vi "Init Actor Core.vi"(8 "error in (no error)":errorcluster, 11 "App in":refnum<class "App.lvclass">) -> (0 "error out":errorcluster, 3 "App out":refnum<class "App.lvclass">)   [LabVIEW 2016, in "App.lvlib" / "App.lvclass"]
uses:
  App.lvclass
  App.lvclass/App.ctl
  Dynamic Instrument/Dynamic Instrument/Dynamic Instrument.lvclass
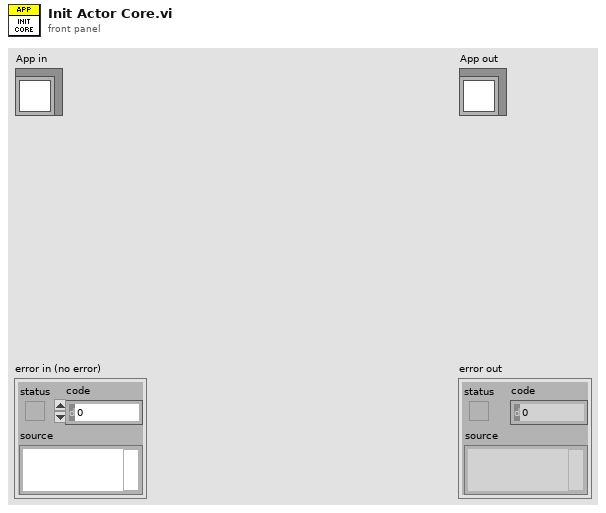
[diagram p1: front panel]
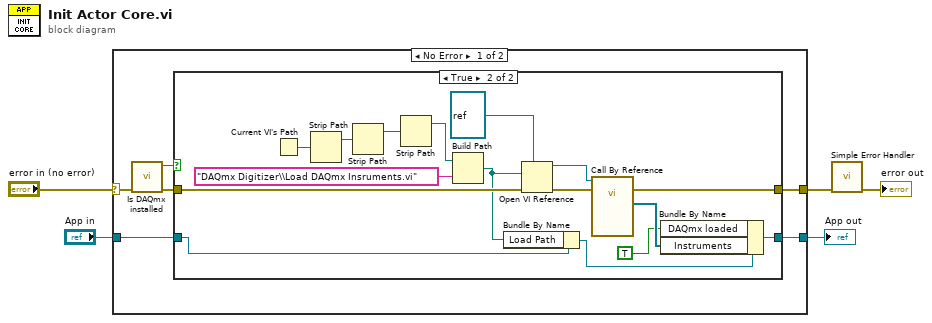
[diagram p0: block diagram]
diagram:
  n1 = case shown="No Error" "error in (no error)" {
    selector: "error in (no error)" -> [w7 w31]
    tunnel: [w9 w31] -> w4
    tunnel: [w10 w30] -> w2
    tunnel: "App in" -> [w11 w30]
    frame No Error {
      n2 = call "Is DAQmx installed.vi"("Error In"=w7) -> ("Error Out"=w6:errorcluster, "file or folder exists?"=w8:bool)  [unwired: 9 in]
      n3 = case shown="True" w8 {
        tunnel: w11 -> [w12 w24]
        tunnel: [w12 w23] -> w10
        tunnel: w6 -> [w13 w22]
        tunnel: [w13 w21] -> w9
        frame False {
        }
        frame True {
          n4 = Current VI's Path() -> (path=w28:path)
          n5 = Strip Path(path=w28) -> (stripped path=w20:path)  [unwired: 1 out]
          n6 = Strip Path(path=w20) -> (stripped path=w16:path)  [unwired: 1 out]
          n7 = Strip Path(path=w16) -> (stripped path=w19:path)  [unwired: 1 out]
          n8 = Build Path(base path=w19, name or relative path="DAQmx Digitizer\\Load DAQmx Insruments.vi") -> (appended path=w17:path)
          n9 = Bundle By Name(cluster=w24, "Load Path"=w17) -> (w18:refnum<class "App.lvclass">)
          n10 = Open VI Reference(type specifier VI Refnum (for type only)=refnum<vi> refnum, vi path=w17, error in (no error)=w22) -> (vi reference=w26:refnum<vi>, error out=w25:errorcluster)  [unwired: 3 in]
          n11 = call-by-ref "?"(reference=w26, error in=w25) -> (error out=w21:errorcluster, "Instruments"=w15:refnum<class "Dynamic Instrument.lvclass">[])  [unwired: 11 in, 1 out]
          n12 = Bundle By Name(cluster=w18, "DAQmx loaded"=TRUE, "Instruments"=w15) -> (w23:refnum<class "App.lvclass">)
        }
      }
    }
    frame Error {
    }
  }
  "App out" <- w2
  n13 = call <vilib>:"Simple Error Handler.vi"("error in (no error)"=w4) -> ("error out"=→"error out":errorcluster)  [unwired: 4 in, 4 out]
